vi "Loop_SM.vi"() -> ()   [LabVIEW 2017]
uses:
  ENUM_SM_State.ctl
  ENUM_SM_Action.ctl
  TypeDef/CLUSTER_CMD_WC_Drive.ctl
  TypeDef/ENUM_WC_Drive_DriveMode.ctl
  TypeDef/CLUSTER_Drive_ACT Loop_VBus Data.ctl
  TypeDef/CLUSTER_X and Y.ctl
  TypeDef/CLUSTER_Drive_ACT Loop_Profile Data.ctl
  TypeDef/CLUSTER_Left and Right.ctl
  TypeDef/ENUM_Drive_ACT Loop_Mode.ctl
  TypeDef/CLUSTER_Drive_HW_SRX_Status.ctl
  TypeDef/CLUSTER_4296_SRX_Status.ctl
  TypeDef/CLUSTER_SRX_Status Data.ctl
  TypeDef/CLUSTER_SRX_Encoder Data.ctl
  TypeDef/CLUSTER_SRX_PWM Data.ctl
  TypeDef/CLUSTER_SRX_Analog Data.ctl
  TypeDef/CLUSTER_SRX_Limit Switch Data.ctl
  TypeDef/CLUSTER_SRX_Profile Data.ctl
  TypeDef/CLUST_Targeting Data.ctl
  TypeDef/CLUST_Cube Data.ctl
  TypeDef/CLUST_Road Navigation Data.ctl
  <vilib>/Rock Robotics/WPI/ThirdParty/Sensors/navX/_TypeDefs/FRIC_navX_DeviceNumbersTypeDef.ctl
  _SHARE ALL/Global Share All/Global_STOP.vi
  Globals/Global_CMD_Drive.vi
  Global_ACT Write_Data Out.vi
  Globals/Global_Vision_Data.vi
  <vilib>/addons/control/pid/pid.llb/PID (DBL).vi
  Global_SM Write_Data Out.vi
  <vilib>/addons/control/pid/NI_PID_pid.lvlib
  VisionHW Folder/VisionHW.lvlib
panel:
  in  "allowence":dbl=15.0 format="%#_13g"
  in  "PID gains Road Follow":T1={"proportional gain (Kc)"=0.01, "integral time (Ti, min)"=0.0, "derivative time (Td, min)"=0.0} {"derivative time (Td, min)" format="%.3f"; "integral time (Ti, min)" format="%.3f"; "proportional gain (Kc)" format="%.8f"}
  in  "PID gains Cube Follow":T1={"proportional gain (Kc)"=0.01, "integral time (Ti, min)"=0.0, "derivative time (Td, min)"=0.0} {"derivative time (Td, min)" format="%.3f"; "integral time (Ti, min)" format="%.3f"; "proportional gain (Kc)" format="%.8f"}
  in  "Degree allowence":dbl=2.0 format="%#_13g"
  in  "PID gains Lock Angle":T1={"proportional gain (Kc)"=0.01, "integral time (Ti, min)"=0.0, "derivative time (Td, min)"=0.0} {"derivative time (Td, min)" format="%.3f"; "integral time (Ti, min)" format="%.3f"; "proportional gain (Kc)" format="%.8f"}
  in  "MAX sensativity":dbl=1.0
  in  "Max RPM":dbl=10000.0
  in  "MIN sensativity":dbl=0.2
  out "Cycle Time (S)":dbl format="%.3g"
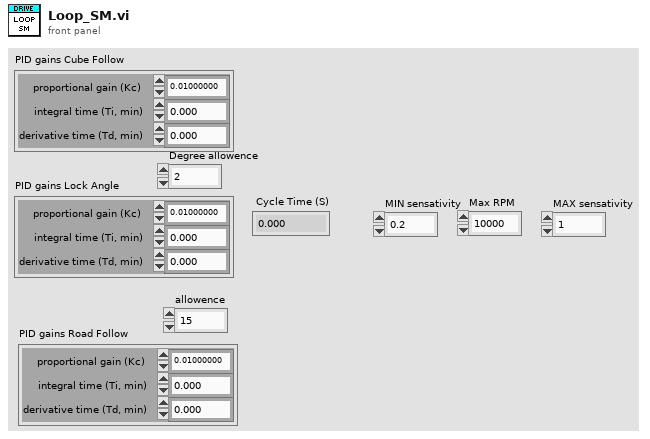
[diagram p1: front panel]
types:
  T1 = cluster{"proportional gain (Kc)":dbl, "integral time (Ti, min)":dbl, "derivative time (Td, min)":dbl}
  T2 = typedef "VisionHW.lvlib/CLUST_Targeting Data.ctl" = cluster{"Cube ":T3, "Road Navigation Data":T4}
  T3 = typedef "VisionHW.lvlib/CLUST_Cube Data.ctl" = cluster{"Height":dbl, "Width":dbl, "Ratio":dbl, "x":i32, "y":i32, "Distance ":i32, "Data Age":dbl}
  T4 = typedef "VisionHW.lvlib/CLUST_Road Navigation Data.ctl" = cluster{"Error":i32, "Data Age":dbl}
  T5 = cluster{"Rollover":dbl, "Yaw":dbl, "Cont Yaw":dbl}
  T6 = typedef "CLUSTER_Drive_HW_SRX_Status.ctl" = cluster{"Rear Left":T7, "Rear Right":T7, "Front Left":T7, "Front Right":T7}
  T7 = typedef "CLUSTER_4296_SRX_Status.ctl" = cluster{"Status":T8, "Encoder":T9, "PWM ":T10, "Analog":T11, "Limit Switches":T12, "Profile":T13}
  T8 = typedef "CLUSTER_SRX_Status Data.ctl" = cluster{"Module Enabled":bool, "Current Profile Slot Select":dbl, "Brake is Enabled":bool, "Applied Throttle":dbl, "Current":dbl, "Battery Voltage":dbl, "Sticky Fault - Under Voltage":bool, "Temperature (C)":dbl, "Sticky Fault - Over Temp":bool, "CAN Error":errorcluster, "Control 5 Is Supported":bool}
  T9 = typedef "CLUSTER_SRX_Encoder Data.ctl" = cluster{"Closed Loop Error":dbl, "Sensor Position":dbl, "Sensor Velocity":dbl, "Encoder Position":dbl, "Encoder Velocity":dbl, "Encoder Index Count":dbl, "Encoder A Pin State":bool, "Encoder B Pin State":bool, "Encoder Index Pin State":bool, "Pos Div 8":bool, "Vel Div 4":bool}
  T10 = typedef "CLUSTER_SRX_PWM Data.ctl" = cluster{"Closed Loop Error":dbl, "Pulse Width Position":i32, "Pulse Width Velocity":i32, "Pulse Width Rise To Rise (us)":i32, "Pulse Width Rise To Fall (us)":i32}
  T11 = typedef "CLUSTER_SRX_Analog Data.ctl" = cluster{"Closed Loop Error":dbl, "Analog In":dbl, "Analog In Velocity":dbl}
  T12 = typedef "CLUSTER_SRX_Limit Switch Data.ctl" = cluster{"Forward Limit Switch Closed":bool, "Reverse Limit Switch Closed":bool, "Sticky Fault - Forward Limit":bool, "Sticky Fault - Reverse Limit":bool, "Sticky Fault - Forward Soft Limit":bool, "Sticky Fault - Reverse Soft Limit":bool}
  T13 = typedef "CLUSTER_SRX_Profile Data.ctl" = cluster{"Mot Prof Active Is Under Run":bool, "Mot Prof Active Has Under Run":bool, "Mot Prof Active Is Last":bool, "Mot Prof Active Velocity Only":bool, "Mot Prof Active Is Valid":bool, "Mot Prof Buffer Is Full":bool, "Mot Prof Active Profile Slot Select":i32, "Mot Prof NextID":i32, "Mot Prof Count":i32, "Mot Prof Active Velocity":dbl, "Mot Prof Active Position":dbl, "Mot Prof Output Enable":i32}
  T14 = typedef "ENUM_Drive_ACT Loop_Mode.ctl" = enum16{"Stop", "Position", "VBus", "Profile"}
  T15 = typedef "CLUSTER_Left and Right.ctl" = cluster{"Left":dbl, "Right":dbl}
  T16 = typedef "CLUSTER_CMD_WC_Drive.ctl" = cluster{"Drive_Mode":T17, "VBus":T18, "Profile":T20, "Zero Drive Encoders":bool, "Set Target Position(IN)":dbl, "Target Angle(Degree)":dbl, "Lock Angle":bool, "Zero YAW":bool, "Follow Cubes":bool, "Follow Road":bool}
  T17 = typedef "ENUM_WC_Drive_DriveMode.ctl" = enum16{"Motion Profile", "CrossLineAuto", "VBus", "Stop"}
  T18 = typedef "CLUSTER_Drive_ACT Loop_VBus Data.ctl" = cluster{"Drive":T19, "Turbo":bool}
  T19 = typedef "CLUSTER_X and Y.ctl" = cluster{"Steer":dbl, "Throtle":dbl}
  T20 = typedef "CLUSTER_Drive_ACT Loop_Profile Data.ctl" = cluster{"Start":bool}
  T21 = typedef "ENUM_SM_Action.ctl" = enum16{"No Action", "Reset Time", "Reset All", "Drive", "Zero YAW", "Shift", "Calculate Sensitivity"}
  T22 = typedef "ENUM_SM_State.ctl" = enum16{"Startup", "VBus", "VBus Lock Angle", "Idle", "Road Follow", "Follow Cube", "Shutdown"}
  T23 = cluster{"Action":T21, "State":T22, "Previous State":T22, "Current Time":timestamp, "Previous Time":timestamp, "Start Time":timestamp, "Target Time (ms)":u32, "Cycle Time(S)":dbl, "CMD_Drive":T16, "VBus Output":T15, "Mode Output":T14, "MQuickStopAccumulator":dbl, "SRX_Status":T6, "Sensitivity":dbl, "NavX Yaw":cluster{"Rollover":dbl, "Yaw":dbl, "Cont Yaw":dbl}, "LockAngle":bool, "Zero YAW":bool, "Target Cube Position (Pixels)":dbl, "Follow Cube":bool, "Follow Road":bool, "Targeting Data":T2}
  T24 = typedef "FRIC_navX_DeviceNumbersTypeDef.ctl" = enum16{"Dev0", "Dev1", "Dev2", "Dev3"}
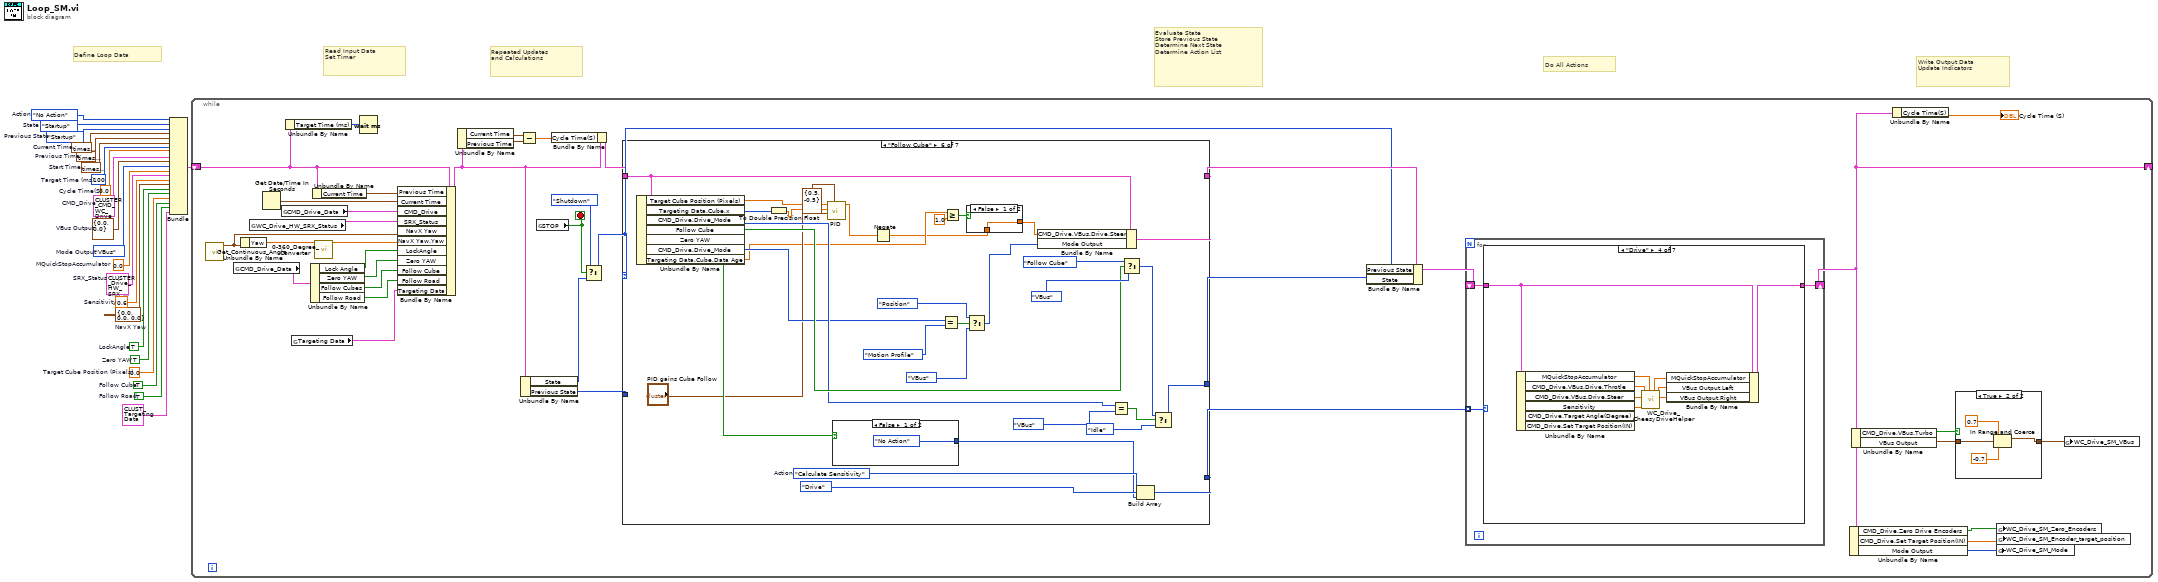
[diagram p0: block diagram]
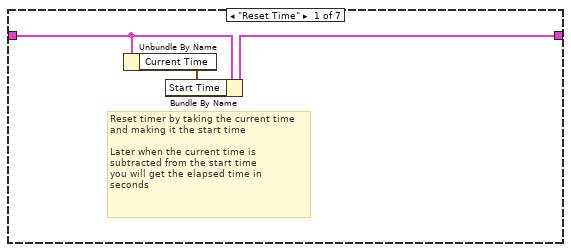
[diagram p3: hidden frame]
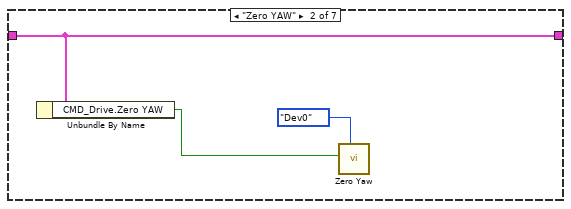
[diagram p4: hidden frame]
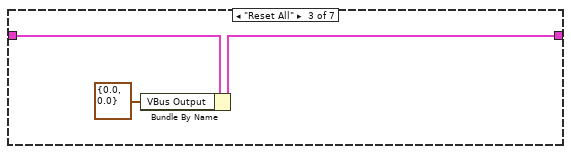
[diagram p5: hidden frame]
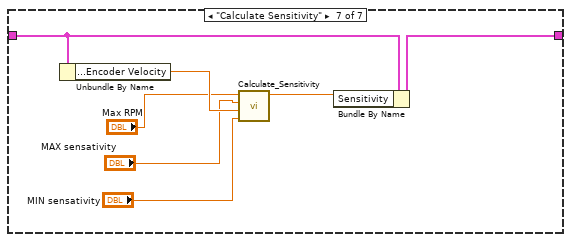
[diagram p8: hidden frame]
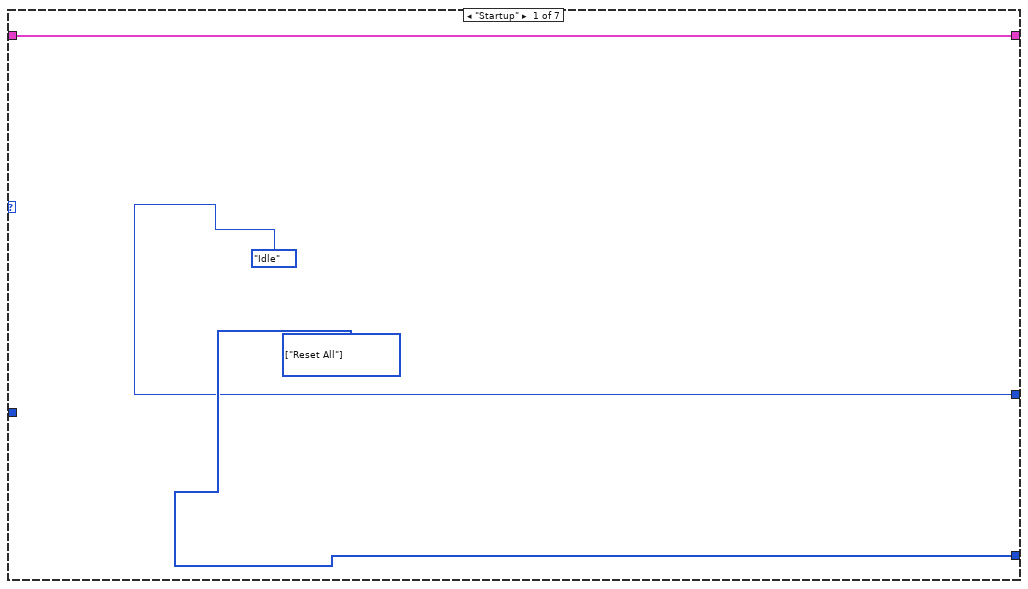
[diagram p9: hidden frame]
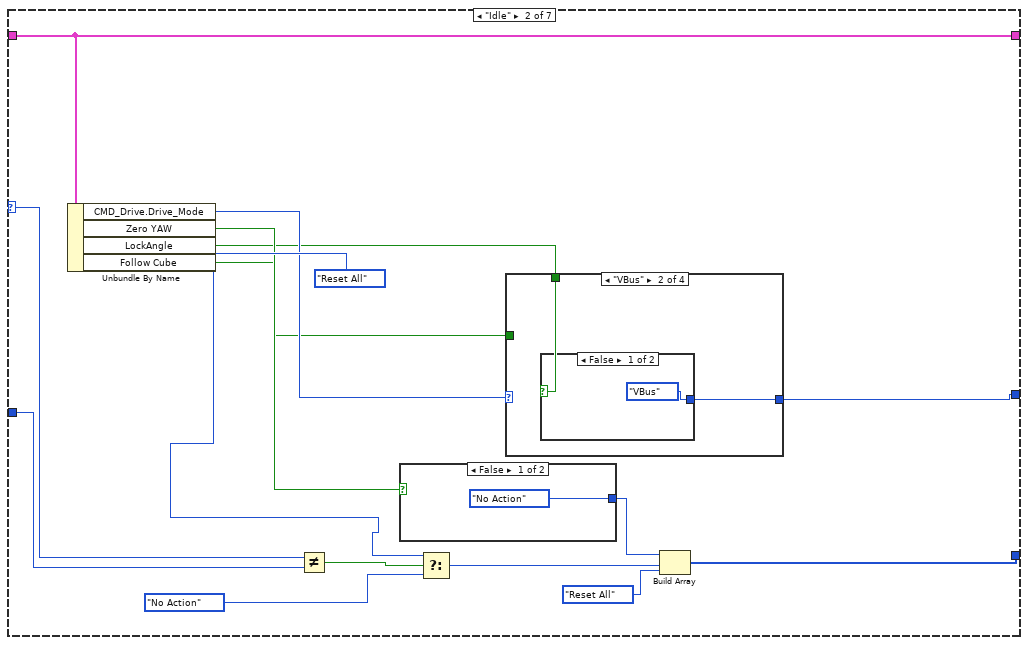
[diagram p10: hidden frame]
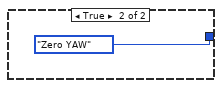
[diagram p11: hidden frame]
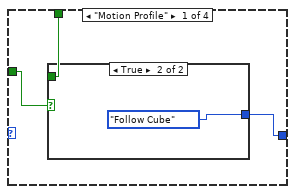
[diagram p12: hidden frame]
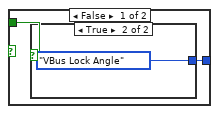
[diagram p13: hidden frame]
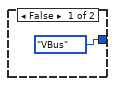
[diagram p14: hidden frame]
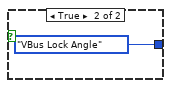
[diagram p15: hidden frame]
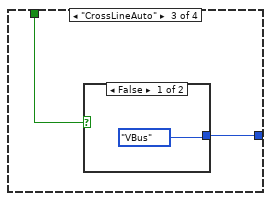
[diagram p16: hidden frame]
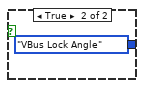
[diagram p17: hidden frame]
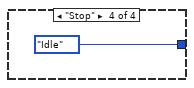
[diagram p18: hidden frame]
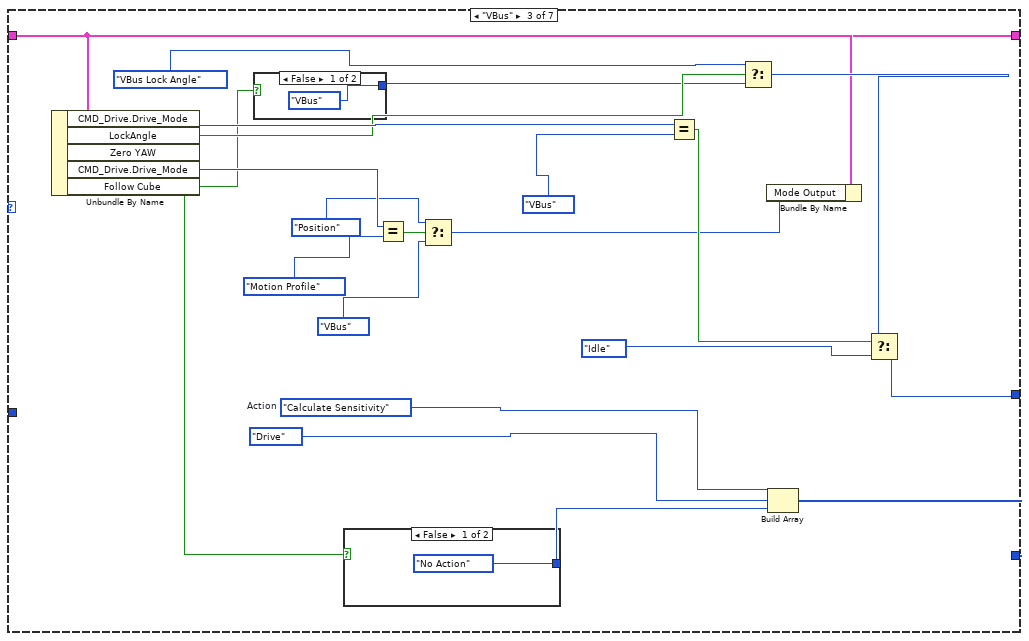
[diagram p19: hidden frame]
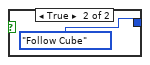
[diagram p20: hidden frame]
diagram:
  w2 = TRUE  # Follow Road
  w3 = TRUE  # Follow Cube
  w4 = 0.0  # Target Cube Position (Pixels)
  w5 = TRUE  # Zero YAW
  w6 = TRUE  # LockAngle
  w7 = T5 {"Rollover"=0.0, "Yaw"=0.0, "Cont Yaw"=0.0}  # NavX Yaw
  w8 = 0.6  # Sensitivity
  w9 = T6 {"Rear Left"={"Status"={"Module Enabled"=FALSE, "Current Profile Slot Select"=0.0, "Brake is Enabled"=TRUE, "Applied Throttle"=0.0, "Current"=0.0, "Battery Voltage"=12.450000000000001, "Sticky Fault - Under Voltage"=TRUE, "Temperature (C)"=30.645161290322577, "Sticky Fault - Over Temp"=FALSE, "CAN Error"={"status"=FALSE, "code"=0, "source"=""}, "Control 5 Is Supported"=TRUE}, "Encoder"={"Closed Loop Error"=0.0, "Sensor Position"=-847.859619140625, "Sensor Velocity"=0.0, "Encoder Position"=-3472833.0, "Encoder Velocity"=0.0, "Encoder Index Count"=-9452.0, "Encoder A Pin State"=FALSE, "Encoder B Pin State"=FALSE, "Encoder Index Pin State"=FALSE, "Pos Div 8"=FALSE, "Vel Div 4"=FALSE}, "PWM "={"Closed Loop Error"=0.0, "Pulse Width Position"=-3472224, "Pulse Width Velocity"=0, "Pulse Width Rise To Rise (us)"=4187, "Pulse Width Rise To Fall (us)"=1210}, "Analog"={"Closed Loop Error"=0.0, "Analog In"=105.0, "Analog In Velocity"=0.0}, "Limit Switches"={"Forward Limit Switch Closed"=FALSE, "Reverse Limit Switch Closed"=FALSE, "Sticky Fault - Forward Limit"=FALSE, "Sticky Fault - Reverse Limit"=TRUE, "Sticky Fault - Forward Soft Limit"=FALSE, "Sticky Fault - Reverse Soft Limit"=FALSE}, "Profile"={"Mot Prof Active Is Under Run"=FALSE, "Mot Prof Active Has Under Run"=FALSE, "Mot Prof Active Is Last"=FALSE, "Mot Prof Active Velocity Only"=FALSE, "Mot Prof Active Is Valid"=FALSE, "Mot Prof Buffer Is Full"=FALSE, "Mot Prof Active Profile Slot Select"=0, "Mot Prof NextID"=0, "Mot Prof Count"=0, "Mot Prof Active Velocity"=0.0, "Mot Prof Active Position"=0.0, "Mot Prof Output Enable"=0}}, "Rear Right"={"Status"={"Module Enabled"=FALSE, "Current Profile Slot Select"=0.0, "Brake is Enabled"=TRUE, "Applied Throttle"=0.0, "Current"=0.125, "Battery Voltage"=12.4, "Sticky Fault - Under Voltage"=TRUE, "Temperature (C)"=27.41935483870968, "Sticky Fault - Over Temp"=FALSE, "CAN Error"={"status"=FALSE, "code"=0, "source"=""}, "Control 5 Is Supported"=TRUE}, "Encoder"={"Closed Loop Error"=0.0, "Sensor Position"=-228.95263671875, "Sensor Velocity"=0.0, "Encoder Position"=937790.0, "Encoder Velocity"=0.0, "Encoder Index Count"=2928.0, "Encoder A Pin State"=FALSE, "Encoder B Pin State"=TRUE, "Encoder Index Pin State"=TRUE, "Pos Div 8"=FALSE, "Vel Div 4"=FALSE}, "PWM "={"Closed Loop Error"=0.0, "Pulse Width Position"=937817, "Pulse Width Velocity"=0, "Pulse Width Rise To Rise (us)"=4128, "Pulse Width Rise To Fall (us)"=3960}, "Analog"={"Closed Loop Error"=0.0, "Analog In"=103.0, "Analog In Velocity"=0.0}, "Limit Switches"={"Forward Limit Switch Closed"=FALSE, "Reverse Limit Switch Closed"=FALSE, "Sticky Fault - Forward Limit"=FALSE, "Sticky Fault - Reverse Limit"=FALSE, "Sticky Fault - Forward Soft Limit"=FALSE, "Sticky Fault - Reverse Soft Limit"=FALSE}, "Profile"={"Mot Prof Active Is Under Run"=FALSE, "Mot Prof Active Has Under Run"=FALSE, "Mot Prof Active Is Last"=FALSE, "Mot Prof Active Velocity Only"=FALSE, "Mot Prof Active Is Valid"=FALSE, "Mot Prof Buffer Is Full"=FALSE, "Mot Prof Active Profile Slot Select"=0, "Mot Prof NextID"=0, "Mot Prof Count"=0, "Mot Prof Active Velocity"=0.0, "Mot Prof Active Position"=0.0, "Mot Prof Output Enable"=0}}, "Front Left"={"Status"={"Module Enabled"=FALSE, "Current Profile Slot Select"=0.0, "Brake is Enabled"=TRUE, "Applied Throttle"=0.0, "Current"=0.0, "Battery Voltage"=12.4, "Sticky Fault - Under Voltage"=TRUE, "Temperature (C)"=28.709677419354833, "Sticky Fault - Over Temp"=FALSE, "CAN Error"={"status"=FALSE, "code"=0, "source"=""}, "Control 5 Is Supported"=TRUE}, "Encoder"={"Closed Loop Error"=0.0, "Sensor Position"=0.0, "Sensor Velocity"=0.0, "Encoder Position"=0.0, "Encoder Velocity"=0.0, "Encoder Index Count"=0.0, "Encoder A Pin State"=TRUE, "Encoder B Pin State"=TRUE, "Encoder Index Pin State"=TRUE, "Pos Div 8"=FALSE, "Vel Div 4"=FALSE}, "PWM "={"Closed Loop Error"=0.0, "Pulse Width Position"=0, "Pulse Width Velocity"=0, "Pulse Width Rise To Rise (us)"=0, "Pulse Width Rise To Fall (us)"=0}, "Analog"={"Closed Loop Error"=0.0, "Analog In"=105.0, "Analog In Velocity"=0.0}, "Limit Switches"={"Forward Limit Switch Closed"=FALSE, "Reverse Limit Switch Closed"=FALSE, "Sticky Fault - Forward Limit"=FALSE, "Sticky Fault - Reverse Limit"=FALSE, "Sticky Fault - Forward Soft Limit"=FALSE, "Sticky Fault - Reverse Soft Limit"=FALSE}, "Profile"={"Mot Prof Active Is Under Run"=FALSE, "Mot Prof Active Has Under Run"=FALSE, "Mot Prof Active Is Last"=FALSE, "Mot Prof Active Velocity Only"=FALSE, "Mot Prof Active Is Valid"=FALSE, "Mot Prof Buffer Is Full"=FALSE, "Mot Prof Active Profile Slot Select"=0, "Mot Prof NextID"=0, "Mot Prof Count"=0, "Mot Prof Active Velocity"=0.0, "Mot Prof Active Position"=0.0, "Mot Prof Output Enable"=0}}, "Front Right"={"Status"={"Module Enabled"=FALSE, "Current Profile Slot Select"=0.0, "Brake is Enabled"=TRUE, "Applied Throttle"=0.0, "Current"=0.0, "Battery Voltage"=12.35, "Sticky Fault - Under Voltage"=TRUE, "Temperature (C)"=26.77419354838709, "Sticky Fault - Over Temp"=FALSE, "CAN Error"={"status"=FALSE, "code"=0, "source"=""}, "Control 5 Is Supported"=TRUE}, "Encoder"={"Closed Loop Error"=0.0, "Sensor Position"=0.0, "Sensor Velocity"=0.0, "Encoder Position"=0.0, "Encoder Velocity"=0.0, "Encoder Index Count"=0.0, "Encoder A Pin State"=TRUE, "Encoder B Pin State"=TRUE, "Encoder Index Pin State"=TRUE, "Pos Div 8"=FALSE, "Vel Div 4"=FALSE}, "PWM "={"Closed Loop Error"=0.0, "Pulse Width Position"=0, "Pulse Width Velocity"=0, "Pulse Width Rise To Rise (us)"=0, "Pulse Width Rise To Fall (us)"=0}, "Analog"={"Closed Loop Error"=0.0, "Analog In"=102.0, "Analog In Velocity"=0.0}, "Limit Switches"={"Forward Limit Switch Closed"=FALSE, "Reverse Limit Switch Closed"=FALSE, "Sticky Fault - Forward Limit"=FALSE, "Sticky Fault - Reverse Limit"=TRUE, "Sticky Fault - Forward Soft Limit"=FALSE, "Sticky Fault - Reverse Soft Limit"=FALSE}, "Profile"={"Mot Prof Active Is Under Run"=FALSE, "Mot Prof Active Has Under Run"=FALSE, "Mot Prof Active Is Last"=FALSE, "Mot Prof Active Velocity Only"=FALSE, "Mot Prof Active Is Valid"=FALSE, "Mot Prof Buffer Is Full"=FALSE, "Mot Prof Active Profile Slot Select"=0, "Mot Prof NextID"=0, "Mot Prof Count"=0, "Mot Prof Active Velocity"=0.0, "Mot Prof Active Position"=0.0, "Mot Prof Output Enable"=0}}}  # SRX_Status
  w10 = 0.0  # MQuickStopAccumulator
  w11 = ENUM_Drive_ACT_Loop_Mode."VBus"  # Mode Output
  w12 = T15 {"Left"=0.0, "Right"=0.0}  # VBus Output
  w13 = T16 {"Drive_Mode"=enum."Motion Profile", "VBus"={"Drive"={"Steer"=0.0, "Throtle"=0.0}, "Turbo"=FALSE}, "Profile"={"Start"=FALSE}, "Zero Drive Encoders"=FALSE, "Set Target Position(IN)"=0.0, "Target Angle(Degree)"=0.0, "Lock Angle"=FALSE, "Zero YAW"=FALSE, "Follow Cubes"=FALSE, "Follow Road"=FALSE}  # CMD_Drive
  w14 = ENUM_SM_Action."No Action"  # Action
  w15 = 0.0  # Cycle Time(S)
  w16 = ENUM_SM_State."Startup"  # Previous State
  w17 = timestamp(0 s since 1904-01-01)  # Previous Time
  w18 = u32 100  # Target Time (ms)
  w19 = timestamp(0 s since 1904-01-01)  # Start Time
  w20 = timestamp(0 s since 1904-01-01)  # Current Time
  w21 = ENUM_SM_State."Startup"  # State
  # "Define Loop Data"
  # "Repeated Updates\nand Calculations"
  # "Read Input Data\nSet Timer"
  # "Evaluate State\nStore Previous State\nDetermine Next State\nDetermine Action List"
  # "Do All Actions"
  # "Write Output Data\nUpdate Indicators"
  n1 = Bundle("Action"=w14, "State"=w21, "Previous State"=w16, "Current Time"=w20, "Previous Time"=w17, "Start Time"=w19, "Target Time (ms)"=w18, "Cycle Time(S)"=w15, "CMD_Drive"=w13, "VBus Output"=w12, "Mode Output"=w11, "MQuickStopAccumulator"=w10, "SRX_Status"=w9, "Sensitivity"=w8, "NavX Yaw"=w7, "LockAngle"=w6, "Zero YAW"=w5, "Target Cube Position (Pixels)"=w4, "Follow Cube"=w3, "Follow Road"=w2, "Targeting Data"=T2 {"Cube "={"Height"=0.0, "Width"=0.0, "Ratio"=0.0, "x"=0, "y"=0, "Distance "=0, "Data Age"=0.0}, "Road Navigation Data"={"Error"=0, "Data Age"=0.0}}) -> (w22:T23)  [unwired: 1 in]
  n2 = while {
    shift-right: [w39] -> _
    shift-left: w22 -> [w50]
    stop <- w55 stop-if-true
    n3 = call <vilib>:"Get_Continuous_Angle.vi"() -> ("Continuous Angle"=w35:T5)  [unwired: 11 in]
    n4 = global read "Global_CMD_Drive.vi" "CMD_Drive_Data"() -> (w30:T16)
    n5 = Unbundle By Name(w35) -> ("Yaw"=w34:dbl)
    n6 = global read "Global_ACT Write_Data Out.vi" "WC_Drive_HW_SRX_Status"() -> (w36:T6)
    n7 = Get Date/Time In Seconds() -> (seconds since 1Jan1904=w59:timestamp)
    n8 = global read "Global_CMD_Drive.vi" "CMD_Drive_Data"() -> (w40:T16)
    n9 = Unbundle By Name(w50) -> ("Target Time (ms)"=w52:u32)
    n10 = global read "Global_Vision_Data.vi" "Targeting Data"() -> (w23:T2)
    n11 = Unbundle By Name(w30) -> ("Lock Angle"=w29:bool, "Zero YAW"=w28:bool, "Follow Cubes"=w25:bool, "Follow Road"=w24:bool)
    n12 = Unbundle By Name(w50) -> ("Current Time"=w51:timestamp)
    n13 = call "0-360_Degree_Converter.vi"("Yaw in"=w34) -> ("Yaw out"=w31:dbl)  [unwired: 10 in]
    n14 = Wait (ms)(milliseconds to wait=w52) -> ()  [unwired: 1 out]
    n15 = Bundle By Name(cluster=w50, "Previous Time"=w51, "Current Time"=w59, "CMD_Drive"=w40, "SRX_Status"=w36, "NavX Yaw"=w35, "NavX Yaw.Yaw"=w31, "LockAngle"=w29, "Zero YAW"=w28, "Follow Cube"=w25, "Follow Road"=w24, "Targeting Data"=w23) -> (w32:T23)
    n16 = Unbundle By Name(w32) -> ("Current Time"=w45:timestamp, "Previous Time"=w46:timestamp)
    n17 = Subtract(x=w45, y=w46) -> (x-y=w43:dbl)
    n18 = Unbundle By Name(w32) -> ("State"=w53:T22, "Previous State"=w49:T22)
    n19 = global read "Global_STOP.vi" "STOP"() -> (w55:bool)
    n20 = Bundle By Name(cluster=w32, "Cycle Time(S)"=w43) -> (w44:T23)
    n21 = Select(t=ENUM_SM_State."Shutdown" ("State"), s=w55, f=w53) -> (s? t:f=w48:T22)
    n22 = case shown="\"Follow Cube\"" w48 {
      selector: w48 -> [_ w106 _ _ _ _ _]
      tunnel: w44 -> [w97 w112 w135 w161 w186 w221 w254]
      tunnel: [w97 w112 w134 w161 w190 w225 w258] -> w57
      tunnel: [ENUM_SM_State."Idle" ("State") w103 w154 ENUM_SM_State."Shutdown" ("State") w178 w214 w247] -> w56
      tunnel: [w96 w107 w150 w159 w187 w222 w255] -> w42
      tunnel: w49 -> [_ w105 _ _ _ _ _]
      frame "Startup" {
        w96 = T21[] [enum."Reset All"] items=["No Action", "Reset Time", "Reset All", "Drive", "Zero YAW", "Shift", "Calculate Sensitivity"] ("Actions")
      }
      frame "Idle" {
        n23 = Unbundle By Name(w112) -> ("CMD_Drive.Drive_Mode"=w104:T17, "Zero YAW"=w101:bool, "LockAngle"=w100:bool, "Follow Cube"=w98:bool)
        n24 = Not Equal?(x=w106, y=w105) -> (x != y?=w111:bool)
        n25 = case shown="False" w101 {
          tunnel: [ENUM_SM_Action."No Action" ("element") ENUM_SM_Action."Zero YAW" ("element")] -> w102
          frame False {
          }
          frame True {
          }
        }
        n26 = Select(t=ENUM_SM_Action."Reset All" ("Action"), s=w111, f=ENUM_SM_Action."No Action" ("Action")) -> (s? t:f=w110:T21)
        n27 = case shown="\"VBus\"" w104 {
          tunnel: [w117 w124 w128 ENUM_SM_State."Idle" ("State")] -> w103
          tunnel: w100 -> [w116 w123 w127 _]
          tunnel: w98 -> [w115 _ _ _]
          frame "Motion Profile" {
            n28 = case shown="True" w115 {
              tunnel: [w119 ENUM_SM_State."Follow Cube" ("State")] -> w117
              tunnel: w116 -> [w118 _]
              frame False {
                n29 = case shown="True" w118 {
                  tunnel: [ENUM_SM_State."VBus" ("State") ENUM_SM_State."VBus Lock Angle" ("State")] -> w119
                  frame False {
                  }
                  frame True {
                  }
                }
              }
              frame True {
              }
            }
          }
          frame "VBus" {
            n30 = case shown="False" w123 {
              tunnel: [ENUM_SM_State."VBus" ("State") ENUM_SM_State."VBus Lock Angle" ("State")] -> w124
              frame False {
              }
              frame True {
              }
            }
          }
          frame "CrossLineAuto" {
            n31 = case shown="False" w127 {
              tunnel: [ENUM_SM_State."VBus" ("State") ENUM_SM_State."VBus Lock Angle" ("State")] -> w128
              frame False {
              }
              frame True {
              }
            }
          }
          frame "Stop" {
          }
        }
        n32 = Build Array(w102, w110, ENUM_SM_Action."Reset All" ("element")) -> (w107:T21[])
      }
      frame "VBus" {
        w151 = ENUM_SM_Action."Calculate Sensitivity"  # Action
        n33 = Unbundle By Name(w135) -> ("CMD_Drive.Drive_Mode"=w153:T17, "LockAngle"=w145:bool, "Zero YAW"=w142:bool, "CMD_Drive.Drive_Mode"=w138:T17, "Follow Cube"=w132:bool)
        n34 = case shown="False" w132 {
          tunnel: [ENUM_SM_State."VBus" ("State") ENUM_SM_State."Follow Cube" ("State")] -> w143
          frame False {
          }
          frame True {
          }
        }
        n35 = case shown="False" w142 {
          tunnel: [ENUM_SM_Action."No Action" ("element") ENUM_SM_Action."Zero YAW" ("element")] -> w141
          frame False {
          }
          frame True {
          }
        }
        n36 = Equal?(x=w138, y=ENUM_WC_Drive_DriveMode."Motion Profile" ("CMD_Drive.Drive_Mode")) -> (x = y?=w140:bool)
        n37 = Select(t=ENUM_Drive_ACT_Loop_Mode."Position" ("WC_Drive_SM_Mode"), s=w140, f=ENUM_Drive_ACT_Loop_Mode."VBus" ("WC_Drive_SM_Mode")) -> (s? t:f=w133:T14)
        n38 = Equal?(x=w153, y=ENUM_WC_Drive_DriveMode."VBus" ("CMD_Drive_Mode")) -> (x = y?=w152:bool)
        n39 = Select(t=ENUM_SM_State."VBus Lock Angle" ("State"), s=w145, f=w143) -> (s? t:f=w146:T22)
        n40 = Bundle By Name(cluster=w135, "Mode Output"=w133) -> (w134:T23)
        n41 = Build Array(w151, ENUM_SM_Action."Drive" ("element"), w141) -> (w150:T21[])
        n42 = Select(t=w146, s=w152, f=ENUM_SM_State."Idle" ("State")) -> (s? t:f=w154:T22)
      }
      frame "Shutdown" {
        w159 = T21[] [enum."Reset All"] items=["No Action", "Reset Time", "Reset All", "Drive", "Zero YAW", "Shift", "Calculate Sensitivity"] ("Actions")
      }
      frame "VBus Lock Angle" {
        w189 = ENUM_SM_Action."Calculate Sensitivity"  # Action
        n43 = Unbundle By Name(w186) -> ("CMD_Drive.Target Angle(Degree)"=w169:dbl, "NavX Yaw.Yaw"=w172:dbl, "CMD_Drive.Drive_Mode"=w176:T17, "LockAngle"=w177:bool, "Zero YAW"=w170:bool, "CMD_Drive.Drive_Mode"=w164:T17)
        n44 = call-poly <vilib>:"PID.vi"("output range"=cluster{"output high":dbl, "output low":dbl} {"output high"=1.0, "output low"=-1.0}, "PID gains"="PID gains Lock Angle", "process variable"=w172, "setpoint"=w169) -> ("output"=w173:dbl)  [unwired: 6 in, 1 out]
        n45 = case shown="False" w170 {
          tunnel: [ENUM_SM_Action."No Action" ("element") ENUM_SM_Action."Zero YAW" ("element")] -> w171
          frame False {
          }
          frame True {
          }
        }
        n46 = call "Steering_converter.vi"("Yaw"=w172, "setpoint"=w169, "output"=w173, "Degree allowence"="Degree allowence") -> ("Steer"=w174:dbl)  [unwired: 7 in]
        n47 = Equal?(x=w164, y=ENUM_WC_Drive_DriveMode."Motion Profile" ("CMD_Drive.Drive_Mode")) -> (x = y?=w168:bool)
        n48 = Select(t=ENUM_Drive_ACT_Loop_Mode."Position" ("WC_Drive_SM_Mode"), s=w168, f=ENUM_Drive_ACT_Loop_Mode."VBus" ("WC_Drive_SM_Mode")) -> (s? t:f=w163:T14)
        n49 = Bundle By Name(cluster=w186, "CMD_Drive.VBus.Drive.Steer"=w174, "Mode Output"=w163) -> (w190:T23)
        n50 = Equal?(x=w176, y=ENUM_WC_Drive_DriveMode."VBus" ("CMD_Drive_Mode")) -> (x = y?=w184:bool)
        n51 = Select(t=ENUM_SM_State."VBus Lock Angle" ("State"), s=w177, f=ENUM_SM_State."VBus" ("State")) -> (s? t:f=w181:T22)
        n52 = Build Array(w189, ENUM_SM_Action."Drive" ("element"), w171) -> (w187:T21[])
        n53 = Select(t=w181, s=w184, f=ENUM_SM_State."Idle" ("State")) -> (s? t:f=w178:T22)
      }
      frame "Follow Cube" {
        w224 = ENUM_SM_Action."Calculate Sensitivity"  # Action
        n54 = Unbundle By Name(w221) -> ("Target Cube Position (Pixels)"=w208:dbl, "Targeting Data.Cube.x"=w200:i32, "CMD_Drive.Drive_Mode"=w212:T17, "Follow Cube"=w213:bool, "Zero YAW"=w209:bool, "CMD_Drive.Drive_Mode"=w203:T17, "Targeting Data.Cube.Data Age"=w198:dbl)
        n55 = To Double Precision Float(number=w200) -> (double precision float=w195:dbl)
        n56 = call-poly <vilib>:"PID.vi"("output range"=cluster{"output high":dbl, "output low":dbl} {"output high"=0.5, "output low"=-0.5}, "PID gains"="PID gains Cube Follow", "process variable"=w195, "setpoint"=w208) -> ("output"=w194:dbl)  [unwired: 6 in, 1 out]
        n57 = case shown="False" w209 {
          tunnel: [ENUM_SM_Action."No Action" ("element") ENUM_SM_Action."Zero YAW" ("element")] -> w210
          frame False {
          }
          frame True {
          }
        }
        n58 = Negate(x=w194) -> (-x=w193:dbl)
        n59 = Equal?(x=w203, y=ENUM_WC_Drive_DriveMode."Motion Profile" ("CMD_Drive.Drive_Mode")) -> (x = y?=w207:bool)
        n60 = Greater Or Equal?(x=w198, y=1.0) -> (x >= y?=w199:bool)
        n61 = case shown="False" w199 {
          tunnel: [w226 0.0 ("CMD_Drive.VBus.Drive.Steer")] -> w196
          tunnel: w193 -> [w226 _]
          frame False {
          }
          frame True {
          }
        }
        n62 = Select(t=ENUM_Drive_ACT_Loop_Mode."Position" ("WC_Drive_SM_Mode"), s=w207, f=ENUM_Drive_ACT_Loop_Mode."VBus" ("WC_Drive_SM_Mode")) -> (s? t:f=w202:T14)
        n63 = Bundle By Name(cluster=w221, "CMD_Drive.VBus.Drive.Steer"=w196, "Mode Output"=w202) -> (w225:T23)
        n64 = Equal?(x=w212, y=ENUM_WC_Drive_DriveMode."VBus" ("CMD_Drive_Mode")) -> (x = y?=w220:bool)
        n65 = Select(t=ENUM_SM_State."Follow Cube" ("State"), s=w213, f=ENUM_SM_State."VBus" ("State")) -> (s? t:f=w217:T22)
        n66 = Build Array(w224, ENUM_SM_Action."Drive" ("element"), w210) -> (w222:T21[])
        n67 = Select(t=w217, s=w220, f=ENUM_SM_State."Idle" ("State")) -> (s? t:f=w214:T22)
      }
      frame "Road Follow" {
        w257 = ENUM_SM_Action."Calculate Sensitivity"  # Action
        n68 = Unbundle By Name(w254) -> ("Target Cube Position (Pixels)"=w238:dbl, "NavX Yaw.Yaw"=w241:dbl, "CMD_Drive.Drive_Mode"=w245:T17, "Follow Cube"=w246:bool, "Zero YAW"=w239:bool, "CMD_Drive.Drive_Mode"=w233:T17)
        n69 = call-poly <vilib>:"PID.vi"("output range"=cluster{"output high":dbl, "output low":dbl} {"output high"=1.0, "output low"=-1.0}, "PID gains"="PID gains Road Follow", "process variable"=w241, "setpoint"=w238) -> ("output"=w242:dbl)  [unwired: 6 in, 1 out]
        n70 = case shown="False" w239 {
          tunnel: [ENUM_SM_Action."No Action" ("element") ENUM_SM_Action."Zero YAW" ("element")] -> w240
          frame False {
          }
          frame True {
          }
        }
        n71 = call "Steering_converter.vi"("Yaw"=w241, "setpoint"=w238, "output"=w242, "Degree allowence"="allowence") -> ("Steer"=w243:dbl)  [unwired: 7 in]
        n72 = Equal?(x=w233, y=ENUM_WC_Drive_DriveMode."Motion Profile" ("CMD_Drive.Drive_Mode")) -> (x = y?=w237:bool)
        n73 = Select(t=ENUM_Drive_ACT_Loop_Mode."Position" ("WC_Drive_SM_Mode"), s=w237, f=ENUM_Drive_ACT_Loop_Mode."VBus" ("WC_Drive_SM_Mode")) -> (s? t:f=w232:T14)
        n74 = Bundle By Name(cluster=w254, "CMD_Drive.VBus.Drive.Steer"=w243, "Mode Output"=w232) -> (w258:T23)
        n75 = Equal?(x=w245, y=ENUM_WC_Drive_DriveMode."VBus" ("CMD_Drive_Mode")) -> (x = y?=w253:bool)
        n76 = Select(t=ENUM_SM_State."Road Follow" ("State"), s=w246, f=ENUM_SM_State."VBus" ("State")) -> (s? t:f=w250:T22)
        n77 = Build Array(w257, ENUM_SM_Action."Drive" ("element"), w240) -> (w255:T21[])
        n78 = Select(t=w250, s=w253, f=ENUM_SM_State."Idle" ("State")) -> (s? t:f=w247:T22)
      }
    }
    n79 = Bundle By Name(cluster=w57, "Previous State"=w48, "State"=w56) -> (w58:T23)
    n80 = for {
      tunnel: w42 -> [w67] mode=indexing
      shift-right: [w66] -> w39
      shift-left: w58 -> [w65]
      n81 = case shown="\"Drive\"" w67 {
        tunnel: w65 -> [w70 w72 w76 w85 w86 w87 w94]
        tunnel: [w69 w72 w75 w84 w86 w87 w93] -> w66
        frame "Reset Time" {
          # "Reset timer by taking the current time\nand making it the start time\n\nLater when the current time is \nsubtracted from the start time\nyou will get the elapsed time in \nseconds"
          n82 = Unbundle By Name(w70) -> ("Current Time"=w68:timestamp)
          n83 = Bundle By Name(cluster=w70, "Start Time"=w68) -> (w69:T23)
        }
        frame "Zero YAW" {
          n84 = Unbundle By Name(w72) -> ("CMD_Drive.Zero YAW"=w71:bool)
          n85 = call <vilib>:"Zero Yaw.vi"("Device Number"=FRIC_navX_DeviceNumbersTypeDef."Dev0", "Zero"=w71) -> ()  [unwired: 10 in]
        }
        frame "Reset All" {
          n86 = Bundle By Name(cluster=w76, "VBus Output"=T15 {"Left"=0.0, "Right"=0.0}) -> (w75:T23)
        }
        frame "Drive" {
          n87 = Unbundle By Name(w85) -> ("MQuickStopAccumulator"=w82:dbl, "CMD_Drive.VBus.Drive.Throtle"=w81:dbl, "CMD_Drive.VBus.Drive.Steer"=w80:dbl, "Sensitivity"=w79:dbl)  [unwired: 2 out]
          n88 = call "WC_Drive_CheesyDriveHelper.vi"("MQuickStopAccumulator"=w82, "KTurnSensitivity"=w79, "Steer"=w80, "Throttle"=w81) -> ("RightPwm Out"=w77:dbl, "LeftPwm Out"=w78:dbl, "MQuickStopAccumulator Out"=w83:dbl)  [unwired: 5 in]
          n89 = Bundle By Name(cluster=w85, "MQuickStopAccumulator"=w83, "VBus Output.Left"=w78, "VBus Output.Right"=w77) -> (w84:T23)
        }
        frame "No Action" {
        }
        frame "Shift" {
        }
        frame "Calculate Sensitivity" {
          n90 = Unbundle By Name(w94) -> ("SRX_Status.Rear Right.Encoder.Encoder Velocity"=w91:dbl)
          n91 = call "Calculate_Sensitivity.vi"("Min Sensitivity"="MIN sensativity", "Current RPM"=w91, "Max Sensitivity"="MAX sensativity", "Max RPM"="Max RPM") -> ("Sensitivity"=w92:dbl)  [unwired: 7 in]
          n92 = Bundle By Name(cluster=w94, "Sensitivity"=w92) -> (w93:T23)
        }
      }
    }
    n93 = Unbundle By Name(w39) -> ("CMD_Drive.Zero Drive Encoders"=w26:bool, "CMD_Drive.Set Target Position(IN)"=w27:dbl, "Mode Output"=w33:T14)
    n94 = Unbundle By Name(w39) -> ("CMD_Drive.VBus.Turbo"=w37:bool, "VBus Output"=w41:T15)
    n95 = Unbundle By Name(w39) -> ("Cycle Time(S)"=→"Cycle Time (S)":dbl)
    n96 = case shown="True" w37 {
      tunnel: w41 -> [w60 w64]
      tunnel: [w60 w61] -> w38
      frame False {
      }
      frame True {
        n97 = In Range and Coerce(upper limit=0.7, x=w64, lower limit=-0.7) -> (coerced(x)=w61:T15)  [unwired: 1 out]
      }
    }
    n98 = global write "Global_SM Write_Data Out.vi" "WC_Drive_SM_Mode"(w33) -> ()
    n99 = global write "Global_SM Write_Data Out.vi" "WC_Drive_SM_Zero_Encoders"(w26) -> ()
    n100 = global write "Global_SM Write_Data Out.vi" "WC_Drive_SM_Encoder_target_position"(w27) -> ()
    n101 = global write "Global_SM Write_Data Out.vi" "WC_Drive_SM_VBus"(w38) -> ()
  }
